vi "Sort 1D Package Version Array.vi"(8 "error in (no error)":errorcluster, 11 "array":string[](array[string])) -> (0 "error out":errorcluster, 3 "sorted array":string[](array[string]))   [LabVIEW 2014, in "NIPM_API.lvlib"]
doc: "Uses the Selection Sort algorithm to sort a 1D array of package versions from lowest to highest version.\n\nINPUT(s)\n<B>Array</B>: This is a 1D string array of package versions\n\nOUTPUT(s)\n<B>Sorted array</B>: Outputs a sorted array of package versions from lowest to highest version"
uses:
  NIPM_API.lvlib
  Version Comparison Operator.ctl
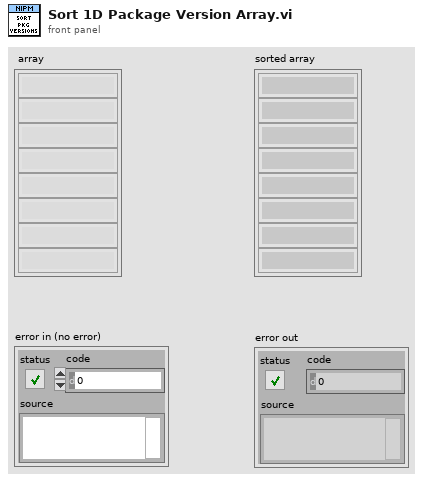
[diagram p1: front panel]
types:
  T1 = typedef "NIPM_API.lvlib/Version Comparison Operator.ctl" = enum16{">", ">=", "=", "!=", "<=", "<"}
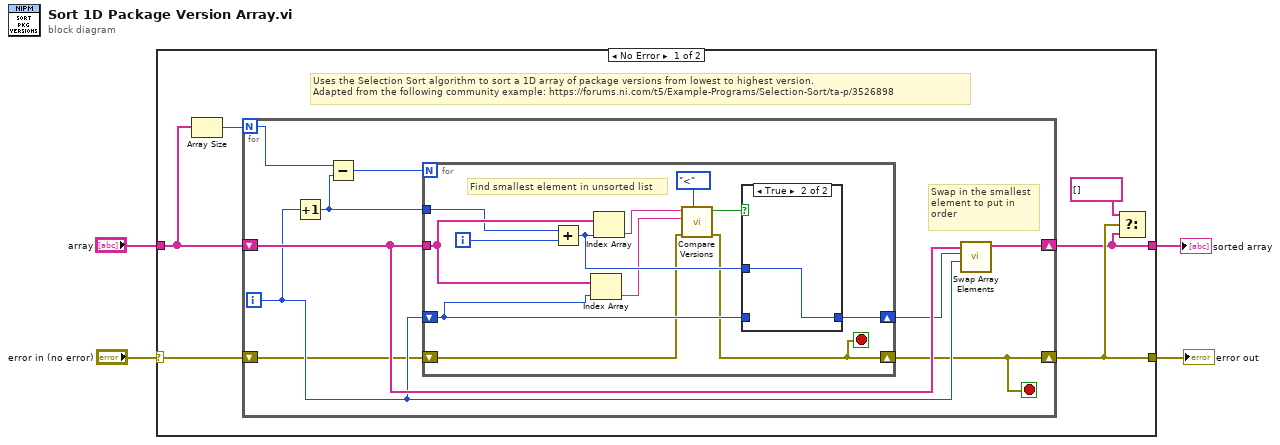
[diagram p0: block diagram]
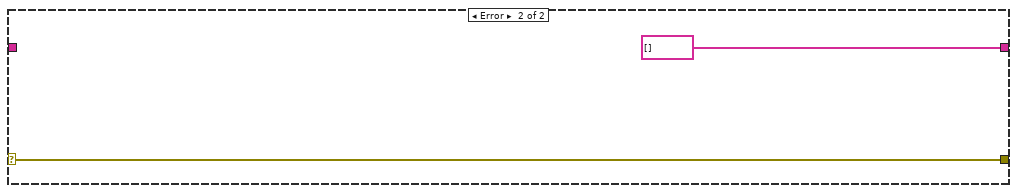
[diagram p3: hidden frame]
diagram:
  n1 = case shown="No Error" "error in (no error)" {
    selector: "error in (no error)" -> [w8 w35]
    tunnel: [w6 string[] [] ("array")] -> w4
    tunnel: "array" -> [w9 _]
    tunnel: [w7 w35] -> w1
    frame No Error {
      # "Uses the Selection Sort algorithm to sort a 1D array of package versions from lowest to highest version.\nAdapted from the following community example: https://forums.ni.com/t5/Example-Programs/Selection-Sort/ta-p/3526898"
      n2 = Array Size(array=w9) -> (size(s)=w10:i32)
      n3 = for {
        N: w10 -> [w16]
        shift-right: [w14] -> w6
        shift-left: w9 -> [w18]
        shift-right: [w11] -> w7
        shift-left: w8 -> [w12]
        i -> [w17]
        stop <- w11 stop-if-true
        # "Swap in the smallest\nelement to put in\norder"
        n4 = Increment(x=w17) -> (x+1=w15:i32)
        n5 = Subtract(x=w16, y=w15) -> (x-y=w19:i32)
        n6 = for {
          N: w19 -> [_]
          tunnel: w18 -> [w30]
          tunnel: w15 -> [w28]
          shift-right: [w22] -> w13
          shift-left: w17 -> [w23]
          shift-right: [w20] -> w11
          shift-left: w12 -> [w21]
          i -> [w29]
          stop <- w20 stop-if-true
          # "Find smallest element in unsorted list"
          n7 = Add(x=w28, y=w29) -> (x+y=w31:i32)
          n8 = Index Array(array=w30, index=w23) -> (element=w25:string)
          n9 = Index Array(array=w30, index=w31) -> (element=w26:string)
          n10 = call "Compare Versions.vi"("operator"=Version_Comparison_Operator."<", "error in"=w21, "version y"=w25, "version x"=w26) -> ("error out"=w20:errorcluster, "Satisfied?"=w24:bool)  [unwired: 6 in]
          n11 = case shown="True" w24 {
            tunnel: w31 -> [_ w33]
            tunnel: w23 -> [w32 _]
            tunnel: [w32 w33] -> w22
            frame False {
            }
            frame True {
            }
          }
        }
        n12 = call "Swap Array Elements.vi"("y"=w17, "x"=w13, "unswapped array"=w18) -> ("swapped array"=w14:string[])  [unwired: 8 in]
      }
      n13 = Select(t=string[] [], s=w7, f=w6) -> ()  [unwired: 1 out]
    }
    frame Error {
    }
  }
  "sorted array" <- w4
  "error out" <- w1
